vi "Get Device Temps.vi"() -> (3 "Device Temperature Data":T1)   [LabVIEW 2015, in "Tool Module.lvlib"]
uses:
  Tool Typedefs/_Temperature All Arrays--typedef.ctl
  ToolModGLOB.vi
  Tool Module.lvlib
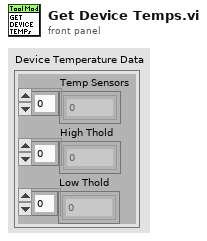
[diagram p1: front panel]
types:
  T1 = typedef "_Temperature All Arrays--typedef.ctl" = cluster{"Temp Sensors":dbl[], "High Thold ":dbl[], "Low Thold ":dbl[]}
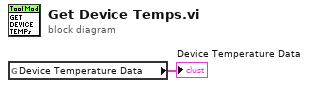
[diagram p0: block diagram]
diagram:
  n1 = global read "ToolModGLOB.vi" "Device Temperature Data"() -> (→"Device Temperature Data":T1)
